vi "Write Meta Data (UDP Clst).vi"(4 "address":cluster{"address":u32, "port":u16}, 6 "options":T3={"ignore timeout error"=TRUE, "timeout ms (1000)"=1000}, 7 "meta data":T2[](array[typedef]), 8 "error in":errorcluster, 11 "connection info in":T1) -> (0 "error out":errorcluster, 3 "connection info out":T1)   [LabVIEW 2010, in "NI STM.lvlib"]
doc: "Use this VI to transmit the meta data cluster to a remote computer. Sending the meta data to another computer helps maintainability since the data resides only on one side and it is shared to other computers at run time."
uses:
  NI STM.lvlib
  SubVIs/MetaDataElement.ctl
  UDP Connection Info.ctl
  UDP Write Options.ctl
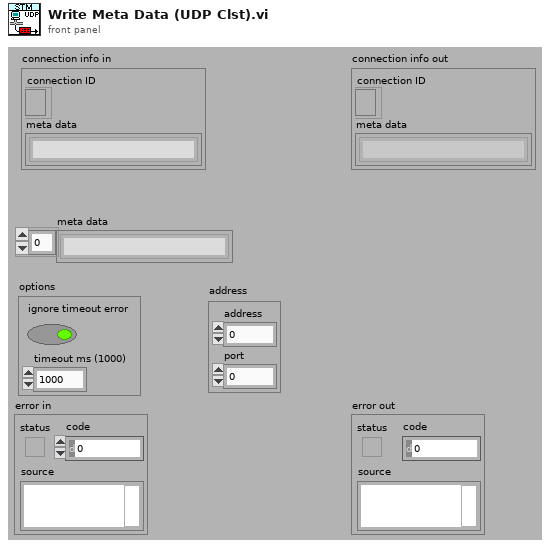
[diagram p1: front panel]
types:
  T1 = typedef "NI STM.lvlib/UDP Connection Info.ctl" = cluster{"connection ID":refnum<k16>, "meta data":T2[]}
  T2 = typedef "NI STM.lvlib/MetaDataElement.ctl" = string
  T3 = typedef "NI STM.lvlib/UDP Write Options.ctl" = cluster{"ignore timeout error":bool, "timeout ms (1000)":i32}
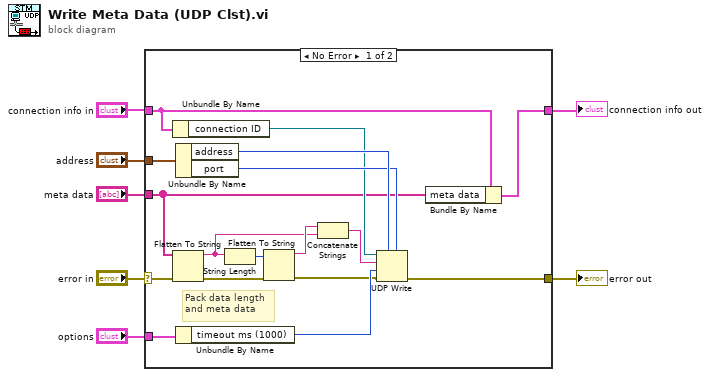
[diagram p0: block diagram]
diagram:
  n1 = case shown="No Error" "error in" {
    selector: "error in" -> [w11 w26]
    tunnel: [w12 w25] -> w7
    tunnel: "connection info in" -> [w13 w25]
    tunnel: "meta data" -> [w8 _]
    tunnel: [w21 w26] -> w5
    tunnel: "address" -> [w19 _]
    tunnel: "options" -> [w16 _]
    frame No Error {
      # "Pack data length\nand meta data"
      n2 = Unbundle By Name(w13) -> ("connection ID"=w14:refnum<k16>)
      n3 = Flatten To String(anything=w8, error in (no error)=w11) -> (data string=w22:string, error out=w10:errorcluster)  [unwired: 3 out]
      n4 = Unbundle By Name(w19) -> ("address"=w18:u32, "port"=w17:u16)
      n5 = Unbundle By Name(w16) -> ("timeout ms (1000)"=w15:i32)
      n6 = String Length(string=w22) -> (length=w24:i32)
      n7 = Flatten To String(anything=w24, error in (no error)=w10) -> (data string=w23:string, error out=w9:errorcluster)  [unwired: 3 out]
      n8 = Concatenate Strings(w23, w22) -> (w20:string)
      n9 = UDP Write(address=w18, port or service name=w17, connection ID=w14, data in=w20, 8:w9, 9:w15) -> (error out=w21:errorcluster)  [unwired: 1 out]
      n10 = Bundle By Name(cluster=w13, "meta data"=w8) -> (w12:T1)
    }
    frame Error {
    }
  }
  "error out" <- w5
  "connection info out" <- w7
